vi "BCU诊断标定.vi"(8 "CAN端口":u16(ring), 9 "设备索引号":u16(ring), 10 "CAN卡类型":u32(ring)=21, 11 "Myindex":dbl=1.0) -> (3 "成功":bool)   [LabVIEW 2013] (continued)
                                n3186 = call "二进制解析-8.6.vi"("索引"=w4312, "数值"=w4313) -> ("低位子数组"=w4310:i32[])  [unwired: 1 in, 2 out]
                                n3187 = Insert Into Array(array=w4311, new element=w4310) -> (w4309:i32[])  [unwired: 1 in]
                                n3188 = case shown="2" w4303 {
                                tunnel: [4 6 5] -> w4304
                                frame 0, Default {
                                }
                                frame 2 {
                                }
                                frame 4 {
                                }
                                }
                                n3189 = Reverse 1D Array(array=w4309) -> (reversed array=w4308:i32[])
                                n3190 = for {
                                N: w4304 -> [_]
                                tunnel: w4308 -> [w4326] mode=indexing
                                tunnel: [w4322] -> w4306 mode=indexing
                                n3191 = Equal To 0?(x=w4326) -> (x = 0?=w4325:bool)
                                n3192 = Select(t="无", s=w4325, f="故障") -> (s? t:f=w4322:string)
                                }
                                n3193 = Insert Into Array(array=w4307, new element=w4306) -> (w4305:string[])  [unwired: 1 in]
                              }
                              n3194 = call "详细故障分解.vi"("名称"=string[] ["自检异常(ee_cpu)", "存储空间满(ee_cpu)", "数据写入失败(ee_cpu)", "数据读取异常(ee_cpu)", "自检异常(ee_ext)", "存储空间满(ee_ext)", "数据写入失败(ee_ext)", "数据读取异常(ee_ext)", "自检异常(flash_ext)", "故障数据存储空间满(flash_ext)", "历史数据存储空间满(flash_ext)", "数据写入失败(flash_ext)", "数据读取失败(flash_ext)", "数据校验异常(flash_ext)", "自检异常(flash_cpu)", "存储空间满(flash_cpu)", "数据写入失败(flash_cpu)", "数据读取异常(flash_cpu)", "应用程序异常(cpu)", "应用程序下载异常(cpu)", "AD模块异常(cpu)", "RAM异常(cpu)", "CPU异常下电(cpu)"], "故障输入口"=w4299) -> ("输出数组"=w4297:string[][])  [unwired: 1 in, 2 out]
                              n3195 = local write "电池故障"(w4297) -> ()
                            }
                            frame 3 {
                              n3196 = for {
                                N: 5 -> [_]
                                tunnel: w4331 -> [w4348]
                                shift-right: [w4335] -> w4329
                                shift-left: string[] [] -> [w4337]
                                i -> [w4334]
                                w4342 = 8 ("索引")
                                w4346 = 2 ("y")
                                n3197 = Multiply(x=w4334, y=w4346) -> (x*y=w4347:i32)
                                n3198 = Array Subset(array=w4348, index=w4347, length=w4346) -> (w4345:u8[])
                                n3199 = Index Array(array=w4345) -> (element #1=w4344:u8, element #2=w4343:u8)  [unwired: 2 in]
                                n3200 = call "二进制解析-8.6.vi"("索引"=w4342, "数值"=w4344) -> ("低位子数组"=w4341:i32[])  [unwired: 1 in, 2 out]
                                n3201 = call "二进制解析-8.6.vi"("索引"=w4342, "数值"=w4343) -> ("低位子数组"=w4340:i32[])  [unwired: 1 in, 2 out]
                                n3202 = Insert Into Array(array=w4341, new element=w4340) -> (w4339:i32[])  [unwired: 1 in]
                                n3203 = Reverse 1D Array(array=w4339) -> (reversed array=w4338:i32[])
                                n3204 = for {
                                N: 6 -> [_]
                                tunnel: w4338 -> [w4353] mode=indexing
                                tunnel: [w4349] -> w4336 mode=indexing
                                n3205 = Equal To 0?(x=w4353) -> (x = 0?=w4352:bool)
                                n3206 = Select(t="无", s=w4352, f="故障") -> (s? t:f=w4349:string)
                                }
                                n3207 = Insert Into Array(array=w4337, new element=w4336) -> (w4335:string[])  [unwired: 1 in]
                              }
                              n3208 = call "详细故障分解.vi"("名称"=string[] ["初始化失败(CAN4)", "发送异常(CAN4)", "接收异常(CAN4)", "总线超时(CAN4)", "BUSOFF(CAN4)", "帧格式(CAN4)", "初始化异常(CAN0)", "发送异常(CAN0)", "接收异常(CAN0)", "总线超时(CAN0)", "BUSOFF(CAN0)", "帧格式(CAN0)", "初始化异常(CAN1)", "发送异常(CAN1)", "接收异常(CAN1)", "总线超时(CAN1)", "BUSOFF(CAN1)", "帧格式(CAN1)", "初始化失败(CAN2)", "发送异常(CAN2)", "接收异常(CAN2)", "总线超时(CAN2)", "BUSOFF(CAN2)", "帧格式(CAN2)", "初始化失败(CAN3)", "发送异常(CAN3)", "接收异常(CAN3)", "总线超时(CAN3)", "BUSOFF(CAN3)", "帧格式(CAN3)"], "故障输入口"=w4329) -> ("输出数组"=w4327:string[][])  [unwired: 1 in, 2 out]
                              n3209 = local write "电池故障"(w4327) -> ()
                            }
                            frame 4 {
                              n3210 = for {
                                N: 1 -> [_]
                                tunnel: w4358 -> [w4375]
                                shift-right: [w4362] -> w4356
                                shift-left: string[] [] -> [w4364]
                                i -> [w4361]
                                w4369 = 8 ("索引")
                                w4373 = 2 ("y")
                                n3211 = Multiply(x=w4361, y=w4373) -> (x*y=w4374:i32)
                                n3212 = Array Subset(array=w4375, index=w4374, length=w4373) -> (w4372:u8[])
                                n3213 = Index Array(array=w4372) -> (element #1=w4371:u8, element #2=w4370:u8)  [unwired: 2 in]
                                n3214 = call "二进制解析-8.6.vi"("索引"=w4369, "数值"=w4371) -> ("低位子数组"=w4368:i32[])  [unwired: 1 in, 2 out]
                                n3215 = call "二进制解析-8.6.vi"("索引"=w4369, "数值"=w4370) -> ("低位子数组"=w4367:i32[])  [unwired: 1 in, 2 out]
                                n3216 = Insert Into Array(array=w4368, new element=w4367) -> (w4366:i32[])  [unwired: 1 in]
                                n3217 = Reverse 1D Array(array=w4366) -> (reversed array=w4365:i32[])
                                n3218 = for {
                                N: 4 -> [_]
                                tunnel: w4365 -> [w4380] mode=indexing
                                tunnel: [w4376] -> w4363 mode=indexing
                                n3219 = Equal To 0?(x=w4380) -> (x = 0?=w4379:bool)
                                n3220 = Select(t="无", s=w4379, f="故障") -> (s? t:f=w4376:string)
                                }
                                n3221 = Insert Into Array(array=w4364, new element=w4363) -> (w4362:string[])  [unwired: 1 in]
                              }
                              n3222 = call "详细故障分解.vi"("名称"=string[] ["通讯协议版本不一致(soft)", "系统不同步(soft)", "软件版本不一致(soft)", "同硬件平台不兼容(soft)"], "故障输入口"=w4356) -> ("输出数组"=w4354:string[][])  [unwired: 1 in, 2 out]
                              n3223 = local write "电池故障"(w4354) -> ()
                            }
                            frame 5 {
                              n3224 = for {
                                N: 2 -> [_]
                                tunnel: w4385 -> [w4402]
                                shift-right: [w4389] -> w4383
                                shift-left: string[] [] -> [w4391]
                                i -> [w4388]
                                w4396 = 8 ("索引")
                                w4400 = 2 ("y")
                                n3225 = Multiply(x=w4388, y=w4400) -> (x*y=w4401:i32)
                                n3226 = Array Subset(array=w4402, index=w4401, length=w4400) -> (w4399:u8[])
                                n3227 = Index Array(array=w4399) -> (element #1=w4398:u8, element #2=w4397:u8)  [unwired: 2 in]
                                n3228 = call "二进制解析-8.6.vi"("索引"=w4396, "数值"=w4398) -> ("低位子数组"=w4395:i32[])  [unwired: 1 in, 2 out]
                                n3229 = call "二进制解析-8.6.vi"("索引"=w4396, "数值"=w4397) -> ("低位子数组"=w4394:i32[])  [unwired: 1 in, 2 out]
                                n3230 = Insert Into Array(array=w4395, new element=w4394) -> (w4393:i32[])  [unwired: 1 in]
                                n3231 = Reverse 1D Array(array=w4393) -> (reversed array=w4392:i32[])
                                n3232 = for {
                                N: 4 -> [_]
                                tunnel: w4392 -> [w4407] mode=indexing
                                tunnel: [w4403] -> w4390 mode=indexing
                                n3233 = Equal To 0?(x=w4407) -> (x = 0?=w4406:bool)
                                n3234 = Select(t="无", s=w4406, f="故障") -> (s? t:f=w4403:string)
                                }
                                n3235 = Insert Into Array(array=w4391, new element=w4390) -> (w4389:string[])  [unwired: 1 in]
                              }
                              n3236 = call "详细故障分解.vi"("名称"=string[] ["初始化失败(RS232)", "发送异常(RS232)", "接收异常(RS232)", "总线超时(RS232)", "初始化失败(RS485)", "发送异常(RS485)", "接收异常(RS485)", "总线超时(RS485)"], "故障输入口"=w4383) -> ("输出数组"=w4381:string[][])  [unwired: 1 in, 2 out]
                              n3237 = local write "电池故障"(w4381) -> ()
                            }
                            frame 6 {
                              n3238 = for {
                                N: 2 -> [_]
                                tunnel: w4412 -> [w4429]
                                shift-right: [w4416] -> w4410
                                shift-left: string[] [] -> [w4418]
                                i -> [w4415]
                                w4423 = 8 ("索引")
                                w4427 = 2 ("y")
                                n3239 = Multiply(x=w4415, y=w4427) -> (x*y=w4428:i32)
                                n3240 = Array Subset(array=w4429, index=w4428, length=w4427) -> (w4426:u8[])
                                n3241 = Index Array(array=w4426) -> (element #1=w4425:u8, element #2=w4424:u8)  [unwired: 2 in]
                                n3242 = call "二进制解析-8.6.vi"("索引"=w4423, "数值"=w4425) -> ("低位子数组"=w4422:i32[])  [unwired: 1 in, 2 out]
                                n3243 = call "二进制解析-8.6.vi"("索引"=w4423, "数值"=w4424) -> ("低位子数组"=w4421:i32[])  [unwired: 1 in, 2 out]
                                n3244 = Insert Into Array(array=w4422, new element=w4421) -> (w4420:i32[])  [unwired: 1 in]
                                n3245 = Reverse 1D Array(array=w4420) -> (reversed array=w4419:i32[])
                                n3246 = for {
                                N: 16 -> [_]
                                tunnel: w4419 -> [w4434] mode=indexing
                                tunnel: [w4430] -> w4417 mode=indexing
                                n3247 = Equal To 0?(x=w4434) -> (x = 0?=w4433:bool)
                                n3248 = Select(t="无", s=w4433, f="故障") -> (s? t:f=w4430:string)
                                }
                                n3249 = Insert Into Array(array=w4418, new element=w4417) -> (w4416:string[])  [unwired: 1 in]
                              }
                              n3250 = call "详细故障分解.vi"("名称"=string[] ["DI1对地短", "DI1对电源短", "DI2对地短", "DI2对电源短", "DI3对地短", "DI3对电源短", "DI4对地短", "DI4对电源短", "DI5对地短", "DI5对电源短", "DI6对地短", "DI6对电源短", "DI7对地短", "DI7对电源短", "DI8对地短", "DI8对电源短", "DO1对地短", "DO1对电源短", "DO2对地短", "DO2对电源短", "DO3对地短", "DO3对电源短", "DO4对地短", "DO4对电源短", "DO5对地短", "DO5对电源短", "DO6对地短", "DO6对电源短", "DO7对地短", "DO7对电源短", "DO8对地短", "DO8对电源短"], "故障输入口"=w4410) -> ("输出数组"=w4408:string[][])  [unwired: 1 in, 2 out]
                              n3251 = local write "电池故障"(w4408) -> ()
                            }
                            frame 7 {
                              n3252 = for {
                                N: 2 -> [_]
                                tunnel: w4439 -> [w4456]
                                shift-right: [w4443] -> w4437
                                shift-left: string[] [] -> [w4445]
                                i -> [w4441]
                                w4450 = 8 ("索引")
                                w4454 = 2 ("y")
                                n3253 = Multiply(x=w4441, y=w4454) -> (x*y=w4455:i32)
                                n3254 = Array Subset(array=w4456, index=w4455, length=w4454) -> (w4453:u8[])
                                n3255 = Index Array(array=w4453) -> (element #1=w4452:u8, element #2=w4451:u8)  [unwired: 2 in]
                                n3256 = call "二进制解析-8.6.vi"("索引"=w4450, "数值"=w4452) -> ("低位子数组"=w4449:i32[])  [unwired: 1 in, 2 out]
                                n3257 = call "二进制解析-8.6.vi"("索引"=w4450, "数值"=w4451) -> ("低位子数组"=w4448:i32[])  [unwired: 1 in, 2 out]
                                n3258 = Insert Into Array(array=w4449, new element=w4448) -> (w4447:i32[])  [unwired: 1 in]
                                n3259 = case shown="1" w4441 {
                                tunnel: [4 6] -> w4442
                                frame 0, Default {
                                }
                                frame 1 {
                                }
                                }
                                n3260 = Reverse 1D Array(array=w4447) -> (reversed array=w4446:i32[])
                                n3261 = for {
                                N: w4442 -> [_]
                                tunnel: w4446 -> [w4463] mode=indexing
                                tunnel: [w4459] -> w4444 mode=indexing
                                n3262 = Equal To 0?(x=w4463) -> (x = 0?=w4462:bool)
                                n3263 = Select(t="无", s=w4462, f="故障") -> (s? t:f=w4459:string)
                                }
                                n3264 = Insert Into Array(array=w4445, new element=w4444) -> (w4443:string[])  [unwired: 1 in]
                              }
                              n3265 = call "详细故障分解.vi"("名称"=string[] ["超时(pre-chg)", "后端开路(pre-chg)", "后端短路(pre-chg)", "预充电回路断开(pre-chg)", "正级继电器驱动故障(relay_driver)", "负级继电器驱动故障(relay_driver)", "预充电继电器驱动故障(relay_driver)", "充电继电器驱动故障(relay_driver)", "风机继电器驱动故障(relay_driver)", "加热继电器驱动故障(relay_driver)"], "故障输入口"=w4437) -> ("输出数组"=w4435:string[][])  [unwired: 1 in, 2 out]
                              n3266 = local write "电池故障"(w4435) -> ()
                            }
                          }
                        }
                        frame True {
                          n3267 = Index Array(array=w4467, index #1=0 ("索引"), index #2=1 ("索引")) -> (element #1=w4470:u8, element #2=w4471:u8)
                          n3268 = Join Numbers(hi=w4470, lo=w4471) -> ((hi.lo)=w4469:u16)
                          n3269 = Number To Hexadecimal String(2:w4469) -> (0:w4468:string)  [unwired: 1 out]
                          n3270 = Concatenate Strings("读取错误，代码： " ("字符串"), "0x" ("字符串"), w4468) -> (w4466:string)
                          n3271 = One Button Dialog(message=w4466, button name ("OK")="是" ("按钮名称（“确定”）")) -> ()  [unwired: 1 out]
                        }
                      }
                      n3272 = local write "消除"(FALSE ("消除")) -> ()
                      n3273 = global write "EV05全局变量1.vi" "流控帧 2"(FALSE ("流控帧 2")) -> ()
                      n3274 = local write "控制1"(FALSE ("控制1")) -> ()
                      n3275 = global write "EV05全局变量1.vi" "写入超时"(TRUE ("写入超时")) -> ()
                    }
                  }
                }
              }
            }
          }
        }
      }
      frame Error {
      }
    }
  }
  n3276 = local write "二维码"(w4) -> ()
  n3277 = call <vilib>:"Close Config Data.vi"("error in (no error)"=w12, "refnum"=w13) -> ("error out"=w5:errorcluster)  [unwired: 8 in, 1 out]
  n3278 = case shown="无错误" w14 {
    tunnel: w5 -> [_ _]
    frame No Error {
      n3279 = case shown="\"全部写入\"" "全部写入" {
        frame "假", Default {
          n3280 = local write "强制终止读写标记"(FALSE ("强制终止读写标记")) -> ()
        }
        frame "单个写入" {
          n3281 = local read "主从选择"() -> (w4483:enum32{"主板", "从板"})
          n3282 = case shown="\"主板\", 默认" w4483 {
            tunnel: [w4494 w4509] -> w4480
            tunnel: [0.0 w4507] -> w4484
            tunnel: [_ w4508] -> w4482
            tunnel: [w4492 _] -> w4481
            frame "主板", Default {
              n3283 = stacked-sequence {
                tunnel: [_ w4506] -> w4492
                frame #0 {
                  n3284 = control-ref of="高压参数"() -> (w4497:refnum<vi>)
                  n3285 = control-ref of="电池信息"() -> (w4498:refnum<vi>)
                  n3286 = control-ref of="一级故障"() -> (w4504:refnum<vi>)
                  n3287 = control-ref of="一级故障 2"() -> (w4502:refnum<vi>)
                  n3288 = control-ref of="一级故障 3"() -> (w4501:refnum<vi>)
                  n3289 = control-ref of="加热控制参数"() -> (w4500:refnum<vi>)
                  n3290 = control-ref of="充电控制参数"() -> (w4499:refnum<vi>)
                  n3291 = control-ref of="项目信息"() -> (w4503:refnum<vi>)
                  n3292 = control-ref of="项目信息2"() -> (w4505:refnum<vi>)
                  n3293 = local read "主板数据"() -> (w4495:T4)
                  n3294 = Bundle(cluster=w4495, "项目信息"=w4503, "一级故障 4"=w4505, "一级故障"=w4504, "一级故障 2"=w4502, "一级故障 3"=w4501, "加热控制参数"=w4500, "充电控制参数"=w4499, "高压参数"=w4497, "电池信息"=w4498) -> (w4496:T4)
                  n3295 = local write "主板数据"(w4496) -> ()
                }
                frame #1 {
                  n3296 = control-ref of="主板数据"() -> (w4506:refnum<vi>)
                }
              }
              n3297 = local read "主板选项"() -> (w4494:string)
            }
            frame "从板" {
              n3298 = stacked-sequence {
                tunnel: [_ w4520] -> w4508
                frame #0 {
                  n3299 = control-ref of="从板号"() -> (w4519:refnum<vi>)
                  n3300 = control-ref of="项目信息 2"() -> (w4518:refnum<vi>)
                  n3301 = control-ref of="均衡参数"() -> (w4513:refnum<vi>)
                  n3302 = control-ref of="加热控制参数"() -> (w4517:refnum<vi>)
                  n3303 = control-ref of="一级故障(从板)"() -> (w4516:refnum<vi>)
                  n3304 = control-ref of="二级故障(从板)"() -> (w4515:refnum<vi>)
                  n3305 = control-ref of="三级故障(从板)"() -> (w4514:refnum<vi>)
                  n3306 = control-ref of="电池组信息"() -> (w4510:refnum<vi>)
                  n3307 = local read "从板信息"() -> (w4511:T2)
                  n3308 = Bundle(cluster=w4511, "从板号"=w4519, "项目信息 2"=w4518, "加热控制参数"=w4517, "一级故障(从板)"=w4516, "二级故障(从板)"=w4515, "三级故障(从板)"=w4514, "电池组信息(从板)"=w4510, "均衡参数"=w4513) -> (w4512:T2)
                  n3309 = local write "从板信息"(w4512) -> ()
                }
                frame #1 {
                  n3310 = control-ref of="从板信息"() -> (w4520:refnum<vi>)
                }
              }
              n3311 = local read "从板选项"() -> (w4509:string)
              n3312 = local read "从板号"() -> (w4507:u8)
            }
          }
          n3313 = local read "从板个数"() -> (w4485:dbl)
          n3314 = local read "快换"() -> (w4486:bool)
          n3315 = call "输入数据解析.vi"("单个参数补充"=w4485, "从板号"=w4484, "主板引用"=w4481, "从板引用"=w4482, "主板选项"=w4480, "枚举"=w4483, "快换"=w4486) -> ("输出数组"=w4490:dbl[][], "数组长度"=w4489:dbl[], "循环次数"=w4479:i32, "命令"=w4488:u32, "名称"=w4478:string[], "命令序号"=w4487:u32[])  [unwired: 2 in, 1 out]
          n3316 = for {
            N: w4479 -> [w4526]
            tunnel: w4490 -> [w4536]
            tunnel: w4489 -> [w4535]
            tunnel: w4488 -> [w4534]
            tunnel: w4487 -> [w4533]
            tunnel: w4484 -> [w4524]
            tunnel: w4480 -> [w4532]
            tunnel: w4478 -> [w4528]
            tunnel: [w4521] -> w4477
            i -> [w4527]
            n3317 = Index Array(array=w4536, index (row)=w4527) -> (element=w4531:dbl[])  [unwired: 1 in]
            n3318 = Index Array(array=w4535, index=w4527) -> (element=w4530:dbl)
            n3319 = Index Array(array=w4528, index=w4527) -> (element=w4525:string)
            n3320 = case shown="\"假\", 默认" w4525 {
              tunnel: [w4538 w4539] -> w4523
              tunnel: w4524 -> [w4538 _]
              tunnel: [TRUE ("确定") w4540] -> w4522
              frame "假", Default {
              }
              frame "从板号" {
                n3321 = call "请输入当前从板板号"() -> ("当前从板板号"=w4539:dbl, "确定"=w4540:bool)  [unwired: 17 in, 1 out]
                n3322 = local write "当前从板板号"(w4539) -> ()
              }
            }
            n3323 = Index Array(array=w4533, index=w4527) -> (element=w4529:u32)
            n3324 = global write "全局 1.vi" "名称"(w4525) -> ()
            n3325 = case shown="真" w4522 {
              tunnel: w4534 -> [_ w4550]
              tunnel: w4532 -> [_ w4549]
              tunnel: w4531 -> [_ w4548]
              tunnel: w4530 -> [_ w4547]
              tunnel: w4529 -> [_ w4546]
              tunnel: w4527 -> [_ w4545]
              tunnel: w4525 -> [_ w4544]
              tunnel: w4526 -> [_ w4543]
              tunnel: w4523 -> [_ w4542]
              tunnel: [_ w4541] -> w4521
              frame False {
                n3326 = call <vilib>:"Unset Busy.vi"() -> ()  [unwired: 11 in, 1 out]
              }
              frame True {
                n3327 = stacked-sequence {
                  seq-local: [_ _ _ w4578 _ _] -> [_ _ _ _ w4587 _]
                  tunnel: w4548 -> [_ _ w4563 _ _ _]
                  tunnel: w4547 -> [_ _ w4562 _ _ _]
                  tunnel: w4550 -> [_ _ w4556 _ _ _]
                  tunnel: w4546 -> [_ _ w4554 _ _ _]
                  tunnel: w4549 -> [_ _ _ _ _ _]
                  tunnel: w4545 -> [_ _ _ _ _ w4598]
                  tunnel: w4544 -> [_ _ _ _ w4586 _]
                  tunnel: w4543 -> [_ _ _ _ _ w4599]
                  tunnel: w4542 -> [_ _ w4555 _ _ _]
                  tunnel: [_ _ _ _ _ w4596] -> w4541
                  frame #0 {
                    w4552 = FALSE ("流控帧")
                    w4551 = TRUE ("流控帧 2")
                    n3328 = call <vilib>:"Set Busy.vi"("disable click? (T)"=w4552) -> ()  [unwired: 3 in, 8 out]
                    n3329 = global write "EV05全局变量1.vi" "读取超时"(w4552) -> ()
                    n3330 = global write "EV05全局变量1.vi" "流控帧"(w4552) -> ()
                    n3331 = local write "消除"(w4551) -> ()
                    n3332 = local write "控制1"(w4551) -> ()
                    n3333 = global write "EV05全局变量1.vi" "流控帧 2"(w4551) -> ()
                    n3334 = local write "写?"(w4551) -> ()
                  }
                  frame #1 {
                    n3335 = Wait Until Next ms Multiple(millisecond multiple=u32 50 ("毫秒倍数")) -> ()  [unwired: 1 out]
                  }
                  frame #2 {
                    n3336 = local read "设备索引号"() -> (w4558:u16)
                    n3337 = local read "CAN卡类型"() -> (w4559:u32)
                    n3338 = Increment(x=w4562) -> (x+1=w4561:dbl)
                    n3339 = local read "CAN端口"() -> (w4557:u16)
                    n3340 = local write "命令"(w4556) -> ()
                    n3341 = local write "命令序号"(w4554) -> ()
                    n3342 = Reshape Array(w4563, w4561) -> (w4560:dbl[])
                    n3343 = stacked-sequence {
                      tunnel: w4560 -> [_ w4577]
                      tunnel: w4559 -> [w4566 w4576]
                      tunnel: w4558 -> [w4565 w4575]
                      tunnel: w4557 -> [w4564 w4574]
                      tunnel: w4556 -> [_ w4573]
                      tunnel: w4555 -> [_ w4572]
                      tunnel: w4554 -> [_ w4571]
                      frame #0 {
                        n3344 = disable-structure shown="禁用" {
                          disable-tunnel: w4566 -> [w4569 _]
                          disable-tunnel: w4565 -> [w4568 _]
                          disable-tunnel: w4564 -> [w4567 _]
                          frame Disabled {
                            n3345 = dll-call lib="PTH1abs FBluewave New EnergySVN_WorkAutoTest_TestStandtrunkAutoTest_TestStandDriverZlgCanBHN01è¯»ååæ°data\nkerneldlls\nusbcan.dll" fn="VCI_ClearBuffer"("DeviceType"=w4569, "DeviceInd"=w4568, "CANInd"=w4567) -> (error out=w4570:errorcluster)  [unwired: 4 in, 4 out]
                            n3346 = call <vilib>:"Clear Errors.vi"("error in (no error)"=w4570) -> ()  [unwired: 6 in, 1 out]
                          }
                          frame Enabled {
                          }
                        }
                      }
                      frame #1 {
                        n3347 = call "多帧发送机制(EV05).vi"("can卡类型"=w4576, "设备索引号"=w4575, "CAN端口"=w4574, "命令"=w4573, "板号"=w4572, "命令序号"=w4571, "输入数据"=w4577) -> ()  [unwired: 2 in, 11 out]
                      }
                    }
                  }
                  frame #3 {
                    n3348 = while {
                      tunnel: [w4580] -> w4578
                      i -> [w4584]
                      stop <- w4581 stop-if-true
                      n3349 = local read "强制终止读写标记"() -> (w4579:bool)
                      n3350 = global read "EV05全局变量1.vi" "读取超时"() -> (w4580:bool)
                      n3351 = Greater Or Equal?(x=w4584, y=30) -> (x >= y?=w4582:bool)
                      n3352 = Wait Until Next ms Multiple(millisecond multiple=u32 100 ("毫秒倍数")) -> ()  [unwired: 1 out]
                      n3353 = Compound Arithmetic op=OR(w4579, w4580, w4582) -> (w4581:bool)
                    }
                  }
                  frame #4 {
                    n3354 = case shown="假" w4587 {
                      tunnel: w4586 -> [w4588 w4594]
                      frame False {
                        n3355 = control-ref of="结果"() -> (w4592:refnum<vi>)
                        n3356 = Concatenate Strings(w4588, "       写入失败" ("字符串")) -> (w4591:string)
                        n3357 = Build Array(w4591) -> (w4590:string[])
                        n3358 = call "表格编辑.vi"("新元素/子数组"=w4590, "活动单元格:单元格背景色"=u32 16740749, "MCListbox引用句柄"=w4592) -> ()  [unwired: 9 out]
                      }
                      frame True {
                        n3359 = case shown="\"从板号\"" w4594 {
                          frame "假", Default {
                          }
                          frame "从板号" {
                            n3360 = local read "从板号"() -> (w4595:u8)
                            n3361 = local write "当前从板板号"(w4595) -> ()
                          }
                        }
                      }
                    }
                    n3362 = call <vilib>:"Unset Busy.vi"() -> ()  [unwired: 2 in, 10 out]
                  }
                  frame #5 {
                    n3363 = Increment(x=w4598) -> (x+1=w4597:i32)
                    n3364 = Equal?(x=w4599, y=w4597) -> (x = y?=w4596:bool)
                    n3365 = case shown="真" w4596 {
                      frame False {
                      }
                      frame True {
                        n3366 = control-ref of="结果"() -> (w4603:refnum<vi>)
                        n3367 = Concatenate Strings("写入完成" ("字符串")) -> (w4602:string)
                        n3368 = Build Array(w4602) -> (w4601:string[])
                        n3369 = call "表格编辑.vi"("新元素/子数组"=w4601, "活动单元格:单元格背景色"=u32 21937, "MCListbox引用句柄"=w4603) -> ()  [unwired: 9 out]
                      }
                    }
                  }
                }
              }
            }
          }
          n3370 = stacked-sequence {
            tunnel: w4477 -> [_]
            frame #0 {
              n3371 = call <vilib>:"Unset Busy.vi"() -> ()  [unwired: 2 in, 10 out]
              n3372 = local write "强制终止读写标记"(FALSE ("强制停止")) -> ()
            }
          }
        }
        frame "全部写入" {
          n3373 = local read "主从选择"() -> (w4611:enum32{"主板", "从板"})
          n3374 = case shown="\"主板\", 默认" w4611 {
            tunnel: [string[] ["项目信息", "一级故障阀值", "二级故障阀值", "三级故障阀值", "加热控制参数", "充电控制参数", "电池信息", "二维码"] string[] ["从板信息", "一级故障阀值", "二级故障阀值", "三级故障阀值", "均衡参数"]] -> w4608
            tunnel: [0.0 ("从板号") w4789] -> w4612
            tunnel: [w4774 _] -> w4610
            tunnel: [_ w4790] -> w4609
            frame "主板", Default {
              n3375 = stacked-sequence {
                tunnel: [_ w4788] -> w4774
                frame #0 {
                  n3376 = control-ref of="电池信息"() -> (w4780:refnum<vi>)
                  n3377 = control-ref of="高压参数"() -> (w4779:refnum<vi>)
                  n3378 = control-ref of="一级故障"() -> (w4782:refnum<vi>)
                  n3379 = control-ref of="一级故障 2"() -> (w4784:refnum<vi>)
                  n3380 = control-ref of="一级故障 3"() -> (w4785:refnum<vi>)
                  n3381 = control-ref of="加热控制参数"() -> (w4786:refnum<vi>)
                  n3382 = control-ref of="充电控制参数"() -> (w4787:refnum<vi>)
                  n3383 = control-ref of="项目信息"() -> (w4783:refnum<vi>)
                  n3384 = control-ref of="项目信息2"() -> (w4781:refnum<vi>)
                  n3385 = local read "主板数据"() -> (w4778:T4)
                  n3386 = Bundle(cluster=w4778, "项目信息"=w4783, "一级故障 4"=w4781, "一级故障"=w4782, "一级故障 2"=w4784, "一级故障 3"=w4785, "加热控制参数"=w4786, "充电控制参数"=w4787, "高压参数"=w4779, "电池信息"=w4780) -> (w4777:T4)
                  n3387 = local write "主板数据"(w4777) -> ()
                }
                frame #1 {
                  n3388 = control-ref of="主板数据"() -> (w4788:refnum<vi>)
                }
              }
              n3389 = local write "失败?"(FALSE ("失败?")) -> ()
            }
            frame "从板" {
              (unwired) "均衡参数"
              n3390 = stacked-sequence {
                tunnel: [_ w4802] -> w4790
                frame #0 {
                  n3391 = control-ref of="从板号"() -> (w4796:refnum<vi>)
                  n3392 = control-ref of="项目信息 2"() -> (w4797:refnum<vi>)
                  n3393 = control-ref of="均衡参数"() -> (w4794:refnum<vi>)
                  n3394 = control-ref of="加热控制参数"() -> (w4798:refnum<vi>)
                  n3395 = control-ref of="一级故障(从板)"() -> (w4799:refnum<vi>)
                  n3396 = control-ref of="二级故障(从板)"() -> (w4800:refnum<vi>)
                  n3397 = control-ref of="三级故障(从板)"() -> (w4801:refnum<vi>)
                  n3398 = control-ref of="电池组信息"() -> (w4795:refnum<vi>)
                  n3399 = local read "从板信息"() -> (w4793:T2)
                  n3400 = Bundle(cluster=w4793, "从板号"=w4796, "项目信息 2"=w4797, "加热控制参数"=w4798, "一级故障(从板)"=w4799, "二级故障(从板)"=w4800, "三级故障(从板)"=w4801, "电池组信息(从板)"=w4795, "均衡参数"=w4794) -> (w4792:T2)
                  n3401 = local write "从板信息"(w4792) -> ()
                }
                frame #1 {
                  n3402 = control-ref of="从板信息"() -> (w4802:refnum<vi>)
                }
              }
              n3403 = local read "从板号"() -> (w4789:u8)
            }
          }
          n3404 = Array Size(array=w4608) -> (size(s)=w4607:i32)
          n3405 = while {
            tunnel: w4608 -> [w4646] mode=indexing
            tunnel: w4611 -> [w4650]
            tunnel: w4612 -> [w4653]
            tunnel: w4610 -> [w4652]
            tunnel: w4609 -> [w4651]
            tunnel: w4607 -> [w4644]
            tunnel: [w4640] -> w4606
            i -> [w4645]
            stop <- w4641 stop-if-true
            n3406 = local read "二维码"() -> (w4639:string)
            n3407 = Increment(x=w4645) -> (x+1=w4643:i32)
            n3408 = local read "从板个数"() -> (w4658:dbl)
            n3409 = local read "快换"() -> (w4649:bool)
            n3410 = Less Or Equal?(x=w4644, y=w4643) -> (x <= y?=w4640:bool)
            n3411 = call "输入数据解析.vi"("单个参数补充"=w4658, "从板号"=w4653, "主板二维码"=w4639, "主板引用"=w4652, "从板引用"=w4651, "主板选项"=w4646, "枚举"=w4650, "快换"=w4649) -> ("输出数组"=w4657:dbl[][], "数组长度"=w4656:dbl[], "循环次数"=w4648:i32, "命令"=w4655:u32, "名称"=w4647:string[], "命令序号"=w4654:u32[])  [unwired: 1 in, 1 out]
            n3412 = case shown="\"主板\", 默认" w4650 {
              tunnel: w4645 -> [w4660 w4674]
              frame "主板", Default {
                n3413 = case shown="6" w4660 {
                  tunnel: [T8."项目信息" ("主从板") T8."一级故障阀值" ("主从板") T8."二级故障阀值" ("主从板") T8."三级故障阀值" ("主从板") T8."控制参数" ("主从板") T8."电池信息" ("主从板")] -> w4659
                  frame 0, Default {
                    n3414 = local write "1"(TRUE ("1")) -> ()
                  }
                  frame 1 {
                    n3415 = local write "1 2"(TRUE ("1 2")) -> ()
                  }
                  frame 2 {
                    n3416 = local write "1 3"(TRUE ("1 3")) -> ()
                  }
                  frame 3 {
                    n3417 = local write "1 4"(TRUE ("1 4")) -> ()
                  }
                  frame 4, 5 {
                    n3418 = local write "1 5"(TRUE ("1 5")) -> ()
                  }
                  frame 6 {
                    n3419 = local write "1 11"(TRUE ("1 11")) -> ()
                  }
                }
                n3420 = local write "主板2"(w4659) -> ()
              }
              frame "从板" {
                n3421 = case shown="1" w4674 {
                  tunnel: [T21."从板信息" ("等级 2") T21."从板信息" ("等级 2") T21."一级故障阀值" ("等级 2") T21."二级故障阀值" ("等级 2") T21."三级故障阀值" ("等级 2") T21."快换参数" ("等级 2") T14."均衡参数" ("等级 2")] -> w4673
                  frame 99, Default {
                    n3422 = local write "1 6"(TRUE ("1 6")) -> ()
                  }
                  frame 0 {
                    n3423 = local write "1 6"(TRUE ("1 6")) -> ()
                  }
                  frame 1 {
                    n3424 = local write "1 7"(TRUE ("1 7")) -> ()
                  }
                  frame 2 {
                    n3425 = local write "1 8"(TRUE ("1 8")) -> ()
                  }
                  frame 3 {
                    n3426 = local write "1 9"(TRUE ("1 9")) -> ()
                  }
                  frame 4 {
                    n3427 = local write "1 10"(TRUE ("1 10")) -> ()
                  }
                  frame 5 {
                    n3428 = local write "1 12"(TRUE ("1 10")) -> ()
                  }
                }
                n3429 = local write "等级 2"(w4673) -> ()
              }
            }
            n3430 = for {
              N: w4648 -> [w4691]
              tunnel: w4657 -> [w4701]
              tunnel: w4656 -> [w4700]
              tunnel: w4655 -> [w4699]
              tunnel: w4654 -> [w4697]
              tunnel: w4653 -> [w4698]
              tunnel: w4647 -> [w4694]
              tunnel: w4640 -> [w4689]
              i -> [w4690]
              n3431 = Index Array(array=w4701, index (row)=w4690) -> (element=w4696:dbl[])  [unwired: 1 in]
              n3432 = Index Array(array=w4700, index=w4690) -> (element=w4695:dbl)
              n3433 = Index Array(array=w4694, index=w4690) -> (element=w4692:string)
              n3434 = Index Array(array=w4697, index=w4690) -> (element=w4693:u32)
              n3435 = while {
                tunnel: w4699 -> [w4711]
                tunnel: w4698 -> [w4710]
                tunnel: w4696 -> [w4709]
                tunnel: w4695 -> [w4708]
                tunnel: w4693 -> [w4707]
                tunnel: w4692 -> [w4706]
                tunnel: w4691 -> [w4705]
                tunnel: w4690 -> [w4704]
                tunnel: w4689 -> [w4703]
                stop <- w4702 stop-if-true
                n3436 = stacked-sequence {
                  seq-local: [_ _ _ w4735 _ _] -> [_ _ _ _ w4744 _]
                  tunnel: w4709 -> [_ _ w4722 _ _ _]
                  tunnel: w4708 -> [_ _ w4721 _ _ _]
                  tunnel: w4711 -> [_ _ w4716 _ _ _]
                  tunnel: w4710 -> [_ _ w4719 _ _ _]
                  tunnel: w4707 -> [_ _ w4717 _ _ _]
                  tunnel: w4706 -> [_ _ w4715 _ w4745 _]
                  tunnel: w4705 -> [_ _ _ _ _ w4767]
                  tunnel: w4704 -> [_ _ _ _ _ w4766]
                  tunnel: w4703 -> [_ _ _ _ _ w4764]
                  tunnel: [_ _ _ _ w4743 _] -> w4702
                  frame #0 {
                    w4712 = FALSE ("流控帧")
                    w4713 = TRUE ("流控帧 2")
                    n3437 = call <vilib>:"Set Busy.vi"("disable click? (T)"=w4712) -> ()  [unwired: 3 in, 8 out]
                    n3438 = global write "EV05全局变量1.vi" "读取超时"(w4712) -> ()
                    n3439 = global write "EV05全局变量1.vi" "流控帧"(w4712) -> ()
                    n3440 = local write "消除"(w4713) -> ()
                    n3441 = local write "控制1"(w4713) -> ()
                    n3442 = global write "EV05全局变量1.vi" "流控帧 2"(w4713) -> ()
                    n3443 = local write "写?"(w4713) -> ()
                    n3444 = local write "读取超时"(w4712) -> ()
                    "流控帧 2" <- w4713
                    "流控帧" <- w4712
                  }
                  frame #1 {
                    n3445 = Wait Until Next ms Multiple(millisecond multiple=u32 50 ("毫秒倍数")) -> ()  [unwired: 1 out]
                  }
                  frame #2 {
                    n3446 = global write "全局 1.vi" "名称"(w4715) -> ()
                    n3447 = local write "命令序号"(w4717) -> ()
                    n3448 = local write "命令"(w4716) -> ()
                    n3449 = local read "设备索引号"() -> (w4724:u16)
                    n3450 = local read "CAN卡类型"() -> (w4725:u32)
                    n3451 = Increment(x=w4721) -> (x+1=w4718:dbl)
                    n3452 = local read "CAN端口"() -> (w4723:u16)
                    n3453 = Reshape Array(w4722, w4718) -> (w4720:dbl[])
                    n3454 = stacked-sequence {
                      tunnel: w4725 -> [_ w4734]
                      tunnel: w4724 -> [_ w4733]
                      tunnel: w4723 -> [_ w4732]
                      tunnel: w4720 -> [_ w4731]
                      tunnel: w4719 -> [_ w4730]
                      tunnel: w4717 -> [_ w4729]
                      tunnel: w4716 -> [_ w4728]
                      frame #0 {
                      }
                      frame #1 {
                        n3455 = control-ref of="流控帧"() -> (w4726:refnum<vi>)
                        n3456 = call "多帧发送机制(EV05).vi"("can卡类型"=w4734, "设备索引号"=w4733, "CAN端口"=w4732, "命令"=w4728, "板号"=w4730, "命令序号"=w4729, "输入数据"=w4731, "流控帧"=w4726) -> ("错误输出"=w4727:errorcluster)  [unwired: 1 in, 10 out]
                        n3457 = call <vilib>:"Clear Errors.vi"("error in (no error)"=w4727) -> ()  [unwired: 6 in, 1 out]
                      }
                    }
                  }
                  frame #3 {
                    n3458 = while {
                      tunnel: [w4736] -> w4735
                      i -> [w4742]
                      stop <- w4739 stop-if-true
                      n3459 = local read "强制终止读写标记"() -> (w4737:bool)
                      n3460 = local read "读取超时"() -> (w4736:bool)
                      n3461 = Greater Or Equal?(x=w4742, y=30) -> (x >= y?=w4740:bool)
                      n3462 = Wait Until Next ms Multiple(millisecond multiple=u32 100 ("毫秒倍数")) -> ()  [unwired: 1 out]
                      n3463 = Compound Arithmetic op=OR(w4737, w4736, w4740) -> (w4739:bool)
                    }
                  }
                  frame #4 {
                    n3464 = case shown="假" w4744 {
                      tunnel: w4745 -> [w4751 _]
                      tunnel: [w4746 TRUE] -> w4743
                      frame False {
                        n3465 = local read "重试次数"() -> (w4750:u8)
                        n3466 = Increment(x=w4750) -> (x+1=w4749:u8)
                        n3467 = Greater Or Equal?(x=w4749, y=u8 4) -> (x >= y?=w4747:bool)
                        n3468 = local write "重试次数"(w4749) -> ()
                        n3469 = case shown="假" w4747 {
                          tunnel: w4751 -> [w4754 _]
                          tunnel: [TRUE FALSE] -> w4746
                          frame False {
                            n3470 = control-ref of="结果"() -> (w4758:refnum<vi>)
                            n3471 = local write "失败?"(TRUE ("失败?")) -> ()
                            n3472 = Concatenate Strings(w4754, "       写入失败" ("字符串")) -> (w4757:string)
                            n3473 = Build Array(w4757) -> (w4756:string[])
                            n3474 = call "表格编辑.vi"("新元素/子数组"=w4756, "活动单元格:单元格背景色"=u32 16740749, "MCListbox引用句柄"=w4758) -> ()  [unwired: 9 out]
                          }
                          frame True {
                          }
                        }
                      }
                      frame True {
                      }
                    }
                  }
                  frame #5 {
                    n3475 = Increment(x=w4766) -> (x+1=w4762:i32)
                    n3476 = Equal?(x=w4767, y=w4762) -> (x = y?=w4765:bool)
                    n3477 = And(x=w4764, y=w4765) -> (x .and. y?=w4763:bool)
                    n3478 = case shown="真" w4763 {
                      frame False {
                      }
                      frame True {
                        n3479 = Concatenate Strings("写入完成" ("字符串")) -> (w4770:string)
                        n3480 = control-ref of="结果"() -> (w4771:refnum<vi>)
                        n3481 = Build Array(w4770) -> (w4769:string[])
                        n3482 = call "表格编辑.vi"("新元素/子数组"=w4769, "活动单元格:单元格背景色"=u32 21937, "MCListbox引用句柄"=w4771) -> ()  [unwired: 9 out]
                      }
                    }
                  }
                }
              }
            }
            n3483 = local read "强制终止读写标记"() -> (w4642:bool)
            n3484 = Or(x=w4640, y=w4642) -> (x .or. y?=w4641:bool)
          }
          n3485 = stacked-sequence {
            tunnel: [_ w4626 _] -> _
            tunnel: w4606 -> [_ _ _]
            frame #0 {
              n3486 = local read "失败?"() -> (w4614:bool)
              n3487 = Not(x=w4614) -> (.not. x?=→"成功":bool)
              n3488 = Select(t="FAIL" ("key"), s=w4614, f="PASS" ("key")) -> (s? t:f=w4617:string)
              n3489 = call <vilib>:"Open Config Data.vi"("error in (no error)"=errorcluster {"status"=FALSE, "code"=0, "source"=""}, "configuration file path"=path "D:/BlueWay/configresult.ini") -> ("error out"=w4623:errorcluster, "refnum"=w4619:T19)  [unwired: 7 in, 1 out]
              n3490 = call-poly <vilib>:"Write Key.vi"("section"="BCURESULT", "error in (no error)"=w4623, "value"=w4617, "key"="BCURESULT", "refnum"=w4619) -> ("error out"=w4624:errorcluster, "refnum out"=w4620:T19)  [unwired: 4 in, 1 out]
              n3491 = call <vilib>:"Close Config Data.vi"("error in (no error)"=w4624, "refnum"=w4620) -> ()  [unwired: 8 in, 2 out]
            }
            frame #1 {
              w4633 = u8 0 items=["Normal", "Listen Only"] ("工作方式")
              w4632 = u8 1 items=["Dual Filter", "Single Filter"] ("滤波方式")
              n3492 = local read "CAN卡类型"() -> (w4627:u32)
              n3493 = local read "设备索引号"() -> (w4628:u16)
              n3494 = local read "CAN端口"() -> (w4629:u16)
              n3495 = call "CAN_Init-8.6.vi"("CAN卡类型"=w4627, "设备索引号"=w4628, "CAN端口"=w4629, "操作类型"=enum16{"初始化CAN", "关闭CAN"}."初始化CAN", "滤波方式"=w4632, "Accept Code"=u32 0, "簇"=T23 {"打开CAN"=FALSE, "初始化CAN"=TRUE, "开始CAN"=TRUE, "重启"=FALSE, "关闭CAN"=FALSE}, "Mask Code"=u32 4294967295 ("Accept Code"), "工作方式"=w4633, "是否滤波"=FALSE, "滤波选择"=T22 {"fiter_mode"=1, "fiter_endid"=0, "fiter_startid"=4294967295}) -> ("error out"=w4626:errorcluster)  [unwired: 3 in, 5 out]
            }
            frame #2 {
              n3496 = local write "停止"(TRUE ("停止")) -> ()
            }
          }
          n3497 = local write "失败?"(FALSE ("失败?")) -> ()
        }
        frame "单个读取" {
          n3498 = stacked-sequence {
            tunnel: [w4805] -> w4803
            frame #0 {
              n3499 = local read "主从选择"() -> (w4806:enum32{"主板", "从板"})
              n3500 = case shown="\"主板\", 默认" w4806 {
                tunnel: [w4819 w4899] -> w4808
                tunnel: [w4818 w4900] -> w4813
                tunnel: [0 ("从板号") w4896] -> w4812
                tunnel: [0 ("板号") u8 0 ("板号")] -> w4811
                tunnel: [w4814 w4895] -> w4809
                frame "主板", Default {
                  n3501 = local read "主板选项"() -> (w4815:string)
                  n3502 = case shown="\"SOC过低(3)\", \"SOC过高(3)\", \"SOH过低(3)\", \"充电电流过高(3)\", \"单体电压过低(3)\", \"单体电压过高(3)\", \"单组电压不均衡(3)\", \"单组温度不均衡(3)\", \"放电电流过高(3)\", \"极柱温度过高(3)\", \"内阻过大(3)\", \"三级故障阀值\", \"温度过低(3)\", \"温度过高(3)\", \"整组电压不均衡(3)\", \"整组温度不均衡(3)\", \"总电压过低(3)\", \"总电压过高(3)\"" w4815 {
                    tunnel: [_ u8[] [1, 2, 3, 4, 5, 6, 13, 8, 7, 9, 10, 11, 12] u8[] [1] u8[] [1] u8[] [2] u8[] [3] u8[] [4] u8[] [5] u8[] [6] u8[] [13] u8[] [7] u8[] [8] u8[] [9] u8[] [10] u8[] [14] u8[] [11] u8[] [12] u8[] [2] u8[] [3] u8[] [1] u8[] [2] u8[] [1] u8[] [2] u8[] [3] u8[] [4] u8[] [1, 2, 3, 4]] -> w4819
                    tunnel: [_ u8 128 ("命令") u8 129 ("命令") u8 128 ("命令") u8 128 ("命令") u8 128 ("命令") u8 128 ("命令") u8 128 ("命令") u8 128 ("命令") u8 128 ("命令") u8 128 ("命令") u8 128 ("命令") u8 128 ("命令") u8 128 ("命令") u8 128 ("命令") u8 128 ("命令") u8 128 ("命令") u8 129 ("命令") u8 129 ("命令") u8 130 ("命令") u8 130 ("命令") u8 132 ("命令") u8 132 ("命令") u8 132 ("命令") u8 132 ("命令") u8 132 ("命令")] -> w4818
                    tunnel: [_ string[] ["产品编号", "电压个数", "通道电压数", "电压起始值", "温度个数", "温度起始值", "保险位置", "电池额定实际容量", "SOC", "配置文件版本", "参数修改记录", "车牌号", "SOH"] string[] ["一级故障阀值"] string[] ["产品编号"] string[] ["电压个数"] string[] ["通道电压数"] string[] ["电压起始值"] string[] ["温度个数"] string[] ["温度起始值"] string[] ["保险位置"] string[] ["SOC"] string[] ["电池额定实际容量"] string[] ["配置文件版本"] string[] ["参数修改记录"] string[] ["校正时钟"] string[] ["车牌号"] string[] ["SOH"] string[] ["二级故障阀值"] string[] ["三级故障阀值"] string[] ["加热控制参数"] string[] ["充电控制参数"] string[] ["电池信息1"] string[] ["电池包组号"] string[] ["充放电安时"] string[] ["电池充放电次数"] string[] ["电池信息1", "电池包组号", "充放电安时", "电池充放电次数"]] -> w4814
                    frame "假", Default {
                    }
                    frame "项目信息" {
                    }
                    frame "SOC过低", "SOC过高", "SOH过低", "充电电流过高", "单体电压过低", "单体电压过高", "单组电压不均衡", "单组温度不均衡", "放电电流过高", "极柱温度过高", "内阻过大", "温度过低", "温度过高", "一级故障阀值", "整组电压不均衡", "整组温度不均衡", "总电压过低", "总电压过高" {
                    }
                    frame "产品编号" {
                    }
                    frame "电压个数" {
                    }
                    frame "通道电压数" {
                    }
                    frame "电压起始值" {
                    }
                    frame "温度个数" {
                    }
                    frame "温度起始值" {
                    }
                    frame "保险位置" {
                    }
                    frame "SOC" {
                    }
                    frame "电池额定实际容量" {
                    }
                    frame "配置文件版本" {
                    }
                    frame "参数修改记录" {
                    }
                    frame "校正时钟" {
                    }
                    frame "车牌号" {
                    }
                    frame "SOH" {
                    }
                    frame "SOC过低(2)", "SOC过高(2)", "SOH过低(2)", "充电电流过高(2)", "单体电压过低(2)", "单体电压过高(2)", "单组电压不均衡(2)", "单组温度不均衡(2)", "二级故障阀值", "放电电流过高(2)", "极柱温度过高(2)", "内阻过大(2)", "温度过低(2)", "温度过高(2)", "整组电压不均衡(2)", "整组温度不均衡(2)", "总电压过低(2)", "总电压过高(2)" {
                    }
                    frame "SOC过低(3)", "SOC过高(3)", "SOH过低(3)", "充电电流过高(3)", "单体电压过低(3)", "单体电压过高(3)", "单组电压不均衡(3)", "单组温度不均衡(3)", "放电电流过高(3)", "极柱温度过高(3)", "内阻过大(3)", "三级故障阀值", "温度过低(3)", "温度过高(3)", "整组电压不均衡(3)", "整组温度不均衡(3)", "总电压过低(3)", "总电压过高(3)" {
                    }
                    frame "风机关闭温差", "风机关闭温度", "风机开启温差", "风机开启温度", "加热关闭温差", "加热关闭温度", "加热开启温度", "加热控制参数" {
                    }
                    frame "充电控制参数", "电流步长", "最大允许充电电流", "最大允许充电温度", "最大允许单体电压", "最大允许总电压", "最小允许充电电流", "最小允许充电温度", "最小允许单体电压" {
                    }
                    frame "电池信息1" {
                    }
                    frame "电池包组号" {
                    }
                    frame "充放电安时" {
                    }
                    frame "电池充放电次数" {
                    }
                    frame "电池信息" {
                    }
                  }
                }
                frame "从板" {
                  n3503 = local read "从板选项"() -> (w4897:string)
                  n3504 = case shown="\"从板信息\"" w4897 {
                    tunnel: [_ u8 0 ("命令") u8 0 ("命令") u8 0 ("命令") u8 0 ("命令") u8 0 ("命令") u8 0 ("命令") u8 0 ("命令") u8 2 ("命令") u8 2 ("命令") u8 2 ("命令") u8 3 ("命令") u8 6 ("命令") u8 6 ("命令") u8 6 ("命令") u8 3 ("命令") u8 3 ("命令") u8 3 ("命令") u8 3 ("命令") u8 3 ("命令") u8 3 ("命令") u8 3 ("命令")] -> w4900
                    tunnel: [_ u8[] [6] u8[] [6, 1, 2, 3, 4, 5] u8[] [1] u8[] [2] u8[] [3] u8[] [4] u8[] [5] u8[] [1] u8[] [2] u8[] [3] u8[] [1, 2, 3, 4, 5, 6, 7] u8[] [1, 2] u8[] [2] u8[] [1] u8[] [1] u8[] [2] u8[] [3] u8[] [4] u8[] [5] u8[] [6] u8[] [7]] -> w4899
                    tunnel: [_ string[] ["从板号"] string[] ["从板号", "电压起始值", "通道电压个数", "保险位置", "温度起始值", "加热控制参数"] string[] ["电压起始值"] string[] ["通道电压节数"] string[] ["保险位置"] string[] ["温度起始值"] string[] ["加热控制参数"] string[] ["一级故障阀值"] string[] ["二级故障阀值"] string[] ["三级故障阀值"] string[] ["电池包信息1", "电池包序号", "充放电安时", "充电次数时间", "SOC", "车牌号", "充电参数"] string[] ["均衡阀值", "充电结束电压"] string[] ["充电结束电压"] string[] ["均衡阀值"] string[] ["电池包信息1"] string[] ["电池包序号"] string[] ["充放电安时"] string[] ["充电次数时间"] string[] ["SOC"] string[] ["车牌号"] string[] ["充电参数"]] -> w4895
                    frame "假", Default {
                    }
                    frame "从板号" {
                    }
                    frame "从板信息" {
                    }
                    frame "电压个数" {
                    }
                    frame "通道电压节数" {
                    }
                    frame "保险位置" {
                    }
                    frame "温度个数" {
                    }
                    frame "风机关闭温差", "风机关闭温度", "风机开启温差", "风机开启温度", "加热关闭温差", "加热关闭温度", "加热开启温度", "加热控制参数" {
                    }
                    frame "SOC过低", "电压不均衡", "电压过低", "电压过高", "温度不均衡", "温度过低", "温度过高", "一级故障阀值" {
                    }
                    frame "SOC过低(2)", "电压不均衡(2)", "电压过低(2)", "电压过高(2)", "二级故障阀值", "温度不均衡(2)", "温度过低(2)", "温度过高(2)" {
                    }
                    frame "SOC过低(3)", "电压不均衡(3)", "电压过低(3)", "电压过高(3)", "三级故障阀值", "温度不均衡(3)", "温度过低(3)", "温度过高(3)" {
                    }
                    frame "快换参数" {
                    }
                    frame "均衡参数" {
                    }
                    frame "充电结束电压" {
                    }
                    frame "均衡阀值" {
                    }
                    frame "电池包信息1" {
                    }
                    frame "电池包序号" {
                    }
                    frame "充放电安时" {
                    }
                    frame "充电次数时间" {
                    }
                    frame "SOC" {
                    }
                    frame "车牌号" {
                    }
                    frame "充电参数" {
                    }
                  }
                  n3505 = local read "从板号"() -> (w4896:u8)
                }
              }
              n3506 = Build Array(w4811) -> (w4810:i32[])
              n3507 = local write "命令"(w4813) -> ()
              n3508 = Array Size(array=w4808) -> (size(s)=w4807:i32)
              n3509 = for {
                tunnel: w4808 -> [w4972] mode=indexing
                tunnel: w4813 -> [w4971]
                tunnel: w4812 -> [w4970]
                tunnel: w4810 -> [w4969]
                tunnel: w4809 -> [w4968] mode=indexing
                tunnel: w4807 -> [w4967]
                tunnel: w4806 -> [w4965]
                tunnel: [w4964] -> w4805
                i -> [w4966]
                n3510 = while {
                  tunnel: w4972 -> [w4981]
                  tunnel: w4971 -> [w4980]
                  tunnel: w4970 -> [w4979]
                  tunnel: w4969 -> [w4978]
                  tunnel: w4968 -> [w4977]
                  tunnel: w4967 -> [w4976]
                  tunnel: w4966 -> [w4975]
                  tunnel: w4965 -> [w4974]
                  tunnel: [w4973] -> w4964
                  stop <- w4973 stop-if-true
                  n3511 = stacked-sequence {
                    seq-local: [_ _ _ _ w5129 _ _] -> [_ _ _ _ _ w5138 _]
                    tunnel: w4981 -> [_ _ _ w5117 _ _ _]
                    tunnel: w4980 -> [_ _ _ w5116 _ _ _]
                    tunnel: w4979 -> [_ _ _ w5115 _ _ _]
                    tunnel: w4978 -> [_ _ _ w5114 _ _ _]
                    tunnel: [_ _ _ _ w5130 _ _] -> w4973
                    tunnel: w4977 -> [w4983 _ _ _ _ w5139 _]
                    tunnel: w4976 -> [_ _ _ _ _ _ w5149]
                    tunnel: w4975 -> [_ _ _ _ _ _ w5148]
                    tunnel: w4974 -> [w4982 _ _ _ _ _ _]
                    frame #0 {
                      n3512 = case shown="\"主板\", 默认" w4982 {
                        tunnel: w4983 -> [w4984 w5075]
                        frame "主板", Default {
                          n3513 = case shown="\"电压个数\"" w4984 {
                            frame "假", Default {
                            }
                            frame "产品编号" {
                              n3514 = control-ref of="产品编号"() -> (w4986:refnum<vi>)
                              n3515 = property class="Str"(reference=w4986, "Value"="") -> ()  [unwired: 1 in, 2 out]
                            }
                            frame "电压个数" {
                              n3516 = local read "从板个数"() -> (w4987:dbl)
                              n3517 = control-ref of="项目信息"() -> (w4991:refnum<vi>)
                              n3518 = for {
                                N: w4987 -> [_]
                                tunnel: [""] -> w4990 mode=indexing
                              }
                              n3519 = call "表格数据输入-8.6.vi"("行数"=u32 0, "列数"=u32 1, "字符串数组"=w4990, "表格引用"=w4991) -> ()  [unwired: 8 in]
                            }
                            frame "通道电压数" {
                              n3520 = control-ref of="项目信息"() -> (w4997:refnum<vi>)
                              n3521 = for {
                                N: 20 -> [_]
                                tunnel: [""] -> w4996 mode=indexing
                              }
                              n3522 = local read "从板个数"() -> (w4998:dbl)
                              n3523 = Increment(x=w4998) -> (x+1=w4994:dbl)
                              n3524 = call "表格数据输入-8.6.vi"("行数"=w4994, "列数"=u32 1, "字符串数组"=w4996, "表格引用"=w4997) -> ()  [unwired: 8 in]
                            }
                            frame "电压起始值" {
                              n3525 = local read "从板个数"() -> (w5002:dbl)
                              n3526 = Increment(x=w5002) -> (x+1=w5001:dbl)
                              n3527 = control-ref of="项目信息"() -> (w5008:refnum<vi>)
                              n3528 = for {
                                N: w5001 -> [_]
                                tunnel: [""] -> w5007 mode=indexing
                              }
                              n3529 = Multiply(x=u8 1, y=w5002) -> (x*y=w5004:dbl)
                              n3530 = Add(x=w5004, y=u8 21) -> (x+y=w5000:dbl)
                              n3531 = call "表格数据输入-8.6.vi"("行数"=w5000, "列数"=u32 1, "字符串数组"=w5007, "表格引用"=w5008) -> ()  [unwired: 8 in]
                            }
                            frame "温度个数" {
                              n3532 = local read "从板个数"() -> (w5012:dbl)
                              n3533 = Increment(x=w5012) -> (x+1=w5011:dbl)
